vi "Dual Stream.vi"() -> ()   [LabVIEW 2016, in "Lab Streaming Layer.lvlib"]
uses:
  Lab Streaming Layer.lvlib
  Custom Controls/lsl_channel_format.ctl
panel:
  out "error out":errorcluster
  out "Array":dbl[][](array[numeric])
  out "Have Consumers":i32
  out "function return":i32
  in  "stop":bool
  out "source id":string
  out "nominal samplerate":dbl
  out "name":string
  out "channel bytes":i32
  out "channel count":i32
  out "xml":string
  out "version":i32
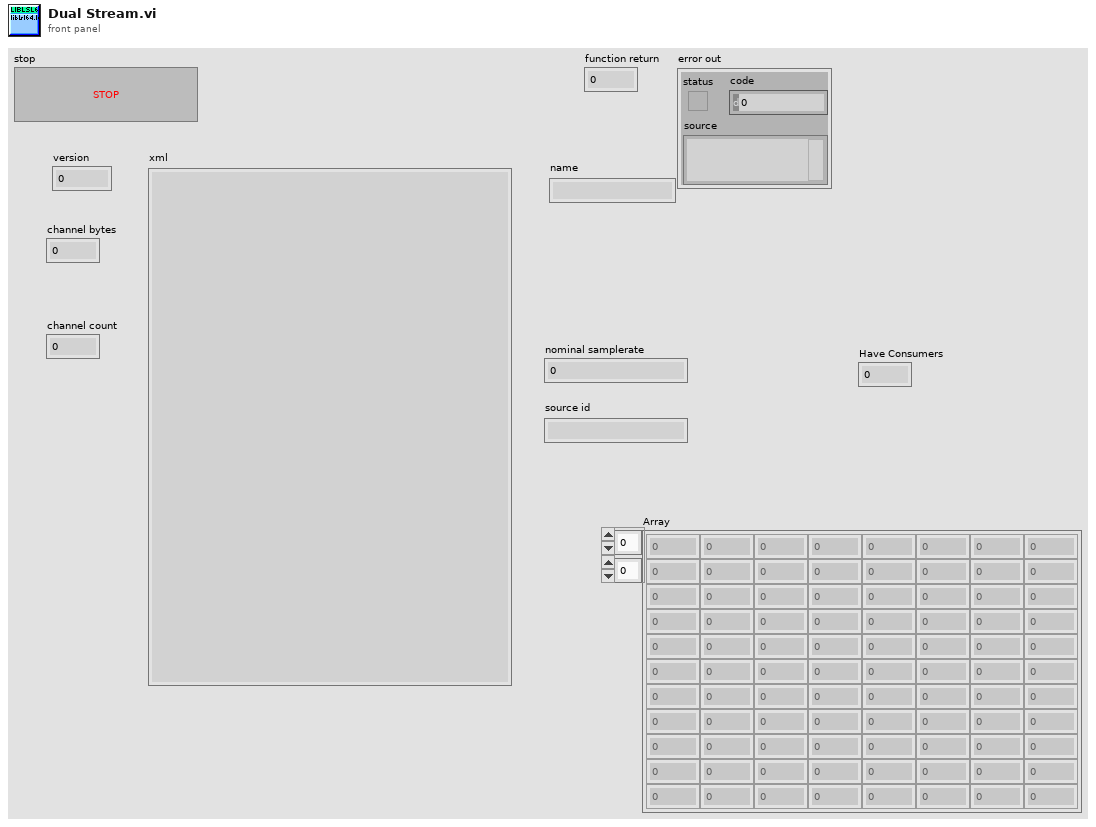
[diagram p1: front panel]
types:
  T1 = typedef "Lab Streaming Layer.lvlib/lsl_channel_format.ctl" = u32
  T2 = typedef "Lab Streaming Layer.lvlib/lsl_streaminfo.ctl" = u64
  T3 = typedef "Lab Streaming Layer.lvlib/lsl_outlet.ctl" = u64
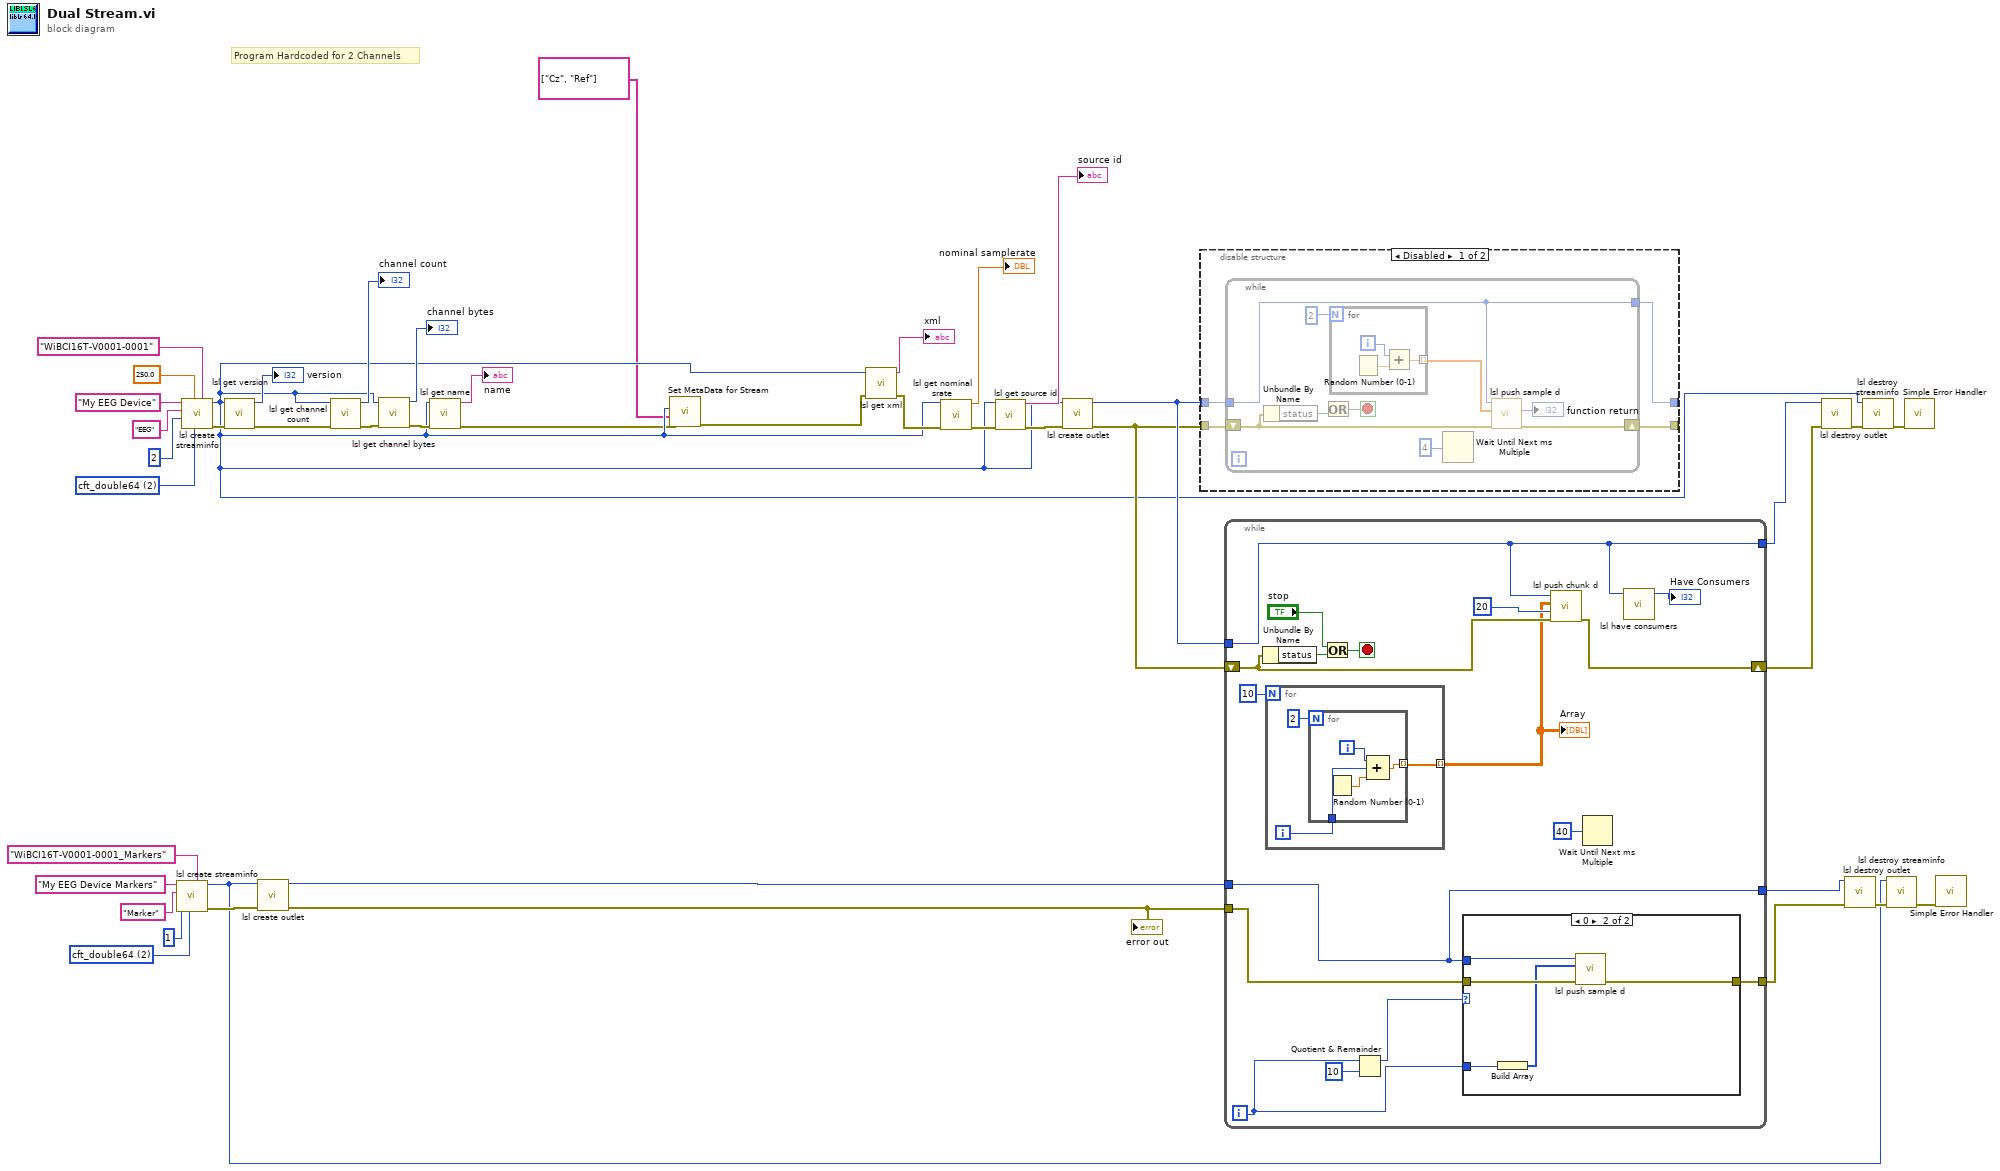
[diagram p0: block diagram]
diagram:
  w10 = T1 2 items=["cft_float32"=1, "cft_double64"=2, "cft_string"=3, "cft_int32"=4, "cft_int16"=5, "cft_int8"=6, "cft_int64"=7, "cft_undefined"=0] ("channel_format")
  w38 = T1 2 items=["cft_float32"=1, "cft_double64"=2, "cft_string"=3, "cft_int32"=4, "cft_int16"=5, "cft_int8"=6, "cft_int64"=7, "cft_undefined"=0] ("channel_format")
  # "Program Hardcoded for 2 Channels"
  n1 = call "lsl create streaminfo.vi"("source_id"="WiBCI16T-V0001-0001_Markers", "channel_format"=w10, "channel_count"=1, "type"="Marker", "name"="My EEG Device Markers") -> ("error out"=w9:errorcluster, "streaminfo"=w2:T2)  [unwired: 5 in]
  n2 = call "lsl create streaminfo.vi"("source_id"="WiBCI16T-V0001-0001", "channel_format"=w38, "samplingrate"=250.0, "channel_count"=2, "type"="EEG", "name"="My EEG Device") -> ("error out"=w37:errorcluster, "streaminfo"=w17:T2)  [unwired: 4 in]
  n3 = call "lsl get version.vi"("error in"=w37, "streaminfo"=w17) -> ("error out"=w20:errorcluster, "version"=→"version":i32)  [unwired: 8 in]
  n4 = call "lsl create outlet.vi"("error in (no error)"=w9, "streaminfo"=w2) -> ("error out"=w7:errorcluster, "outlet"=w8:T3)  [unwired: 8 in]
  "error out" <- w7
  n5 = call "lsl get channel count.vi"("error in (no error)"=w20, "streaminfo"=w17) -> ("error out"=w34:errorcluster, "channel count"=→"channel count":i32)  [unwired: 8 in]
  n6 = call "lsl get channel bytes.vi"("error in (no error)"=w34, "streaminfo"=w17) -> ("error out"=w32:errorcluster, "channel bytes"=→"channel bytes":i32)  [unwired: 8 in]
  n7 = call "lsl get name.vi"("error in (no error)"=w32, "streaminfo"=w17) -> ("error out"=w15:errorcluster, "name"=→"name":string)  [unwired: 8 in]
  n8 = call "Set MetaData for Stream.vi"("error in"=w15, "Ch Names"=string[] ["Cz", "Ref"], "streaminfo"=w17) -> ("error out"=w14:errorcluster)  [unwired: 8 in]
  n9 = call "lsl get xml.vi"("error in (no error)"=w14, "streaminfo"=w17) -> ("error out"=w18:errorcluster, "xml"=→"xml":string)  [unwired: 8 in]
  n10 = call "lsl get nominal srate.vi"("error in (no error)"=w18, "streaminfo"=w17) -> ("error out"=w29:errorcluster, "nominal samplerate"=→"nominal samplerate":dbl)  [unwired: 8 in]
  n11 = call "lsl get source id.vi"("error in (no error)"=w29, "streaminfo"=w17) -> ("error out"=w27:errorcluster, "source id"=→"source id":string)  [unwired: 8 in]
  n12 = call "lsl create outlet.vi"("error in (no error)"=w27, "streaminfo"=w17) -> ("error out"=w23:errorcluster, "outlet"=w24:T3)  [unwired: 8 in]
  n13 = disable-structure shown="Disabled" {
    disable-tunnel: w24 -> [w47 _]
    disable-tunnel: w23 -> [w46 _]
    disable-tunnel: [w45 _] -> _
    disable-tunnel: [w44 _] -> _
    frame Disabled {
      n14 = while {
        tunnel: w47 -> [w48]
        shift-right: [w52] -> w44
        shift-left: w46 -> [w53]
        tunnel: [w48] -> w45
        stop <- w54 stop-if-true
        n15 = Unbundle By Name(w53) -> ("status"=w55:bool)
        n16 = Or(y=w55) -> (x .or. y?=w54:bool)  [unwired: 1 in]
        n17 = for {
          N: 2 -> [_]
          tunnel: [w58] -> w51 mode=indexing
          i -> [w57]
          n18 = Random Number (0-1)() -> (number: 0 to 1=w59:dbl)
          n19 = Add(x=w57, y=w59) -> (x+y=w58:dbl)
        }
        n20 = Wait Until Next ms Multiple(millisecond multiple=u32 4) -> ()  [unwired: 1 out]
        n21 = call "lsl push sample d.vi"("error in (no error)"=w53, "data"=w51, "outlet"=w48) -> ("error out"=w52:errorcluster, "function return"=→"function return":i32)  [unwired: 7 in]
      }
    }
    frame Enabled {
    }
  }
  n22 = while {
    tunnel: w24 -> [w67]
    shift-right: [w72] -> w21
    shift-left: w23 -> [w73]
    tunnel: [w67] -> w22
    tunnel: w8 -> [w61]
    tunnel: w7 -> [w63]
    tunnel: [w61] -> w5
    tunnel: [w60] -> w4
    i -> [w62]
    stop <- w75 stop-if-true
    n23 = Unbundle By Name(w73) -> ("status"=w76:bool)
    n24 = for {
      N: 10 -> [_]
      tunnel: [w84] -> w68 mode=indexing
      i -> [w83]
      n25 = for {
        N: 2 -> [_]
        tunnel: [w89] -> w84 mode=indexing
        tunnel: w83 -> [w87]
        i -> [w88]
        n26 = Random Number (0-1)() -> (number: 0 to 1=w86:dbl)
        n27 = Compound Arithmetic op=ADD(w88, w87, w86) -> (w89:dbl)
      }
    }
    "Array" <- w68
    n28 = Or(x="stop", y=w76) -> (x .or. y?=w75:bool)
    n29 = Quotient & Remainder(x=w62, y=10) -> (x-y*floor(x/y)=w64:i32)  [unwired: 1 out]
    n30 = case shown="0" w64 {
      tunnel: w63 -> [w77 w81]
      tunnel: w61 -> [_ w82]
      tunnel: w62 -> [_ w80]
      tunnel: [w77 w78] -> w60
      frame 1, Default {
      }
      frame 0 {
        n31 = Build Array(w80) -> (w79:i32[])
        n32 = call "lsl push sample d.vi"("error in (no error)"=w81, "data"=w79, "outlet"=w82) -> ("error out"=w78:errorcluster)  [unwired: 7 in, 1 out]
      }
    }
    n33 = call "lsl push chunk d.vi"("error in (no error)"=w73, "data_elements"=i64 20, "data"=w68, "outlet"=w67) -> ("error out"=w72:errorcluster)  [unwired: 6 in, 1 out]
    n34 = Wait Until Next ms Multiple(millisecond multiple=u32 40) -> ()  [unwired: 1 out]
    n35 = call "lsl have consumers.vi"("outlet"=w67) -> ("Have Consumers"=→"Have Consumers":i32)  [unwired: 9 in, 1 out]
  }
  n36 = call "lsl destroy outlet.vi"("error in (no error)"=w21, "outlet"=w22) -> ("error out"=w25:errorcluster)  [unwired: 9 in]
  n37 = call "lsl destroy outlet.vi"("error in (no error)"=w4, "outlet"=w5) -> ("error out"=w6:errorcluster)  [unwired: 9 in]
  n38 = call "lsl destroy streaminfo.vi"("error in (no error)"=w25, "streaminfo"=w17) -> ("error out"=w26:errorcluster)  [unwired: 9 in]
  n39 = call "lsl destroy streaminfo.vi"("error in (no error)"=w6, "streaminfo"=w2) -> ("error out"=w3:errorcluster)  [unwired: 9 in]
  n40 = call <vilib>:"Simple Error Handler.vi"("error in (no error)"=w26) -> ()  [unwired: 4 in, 5 out]
  n41 = call <vilib>:"Simple Error Handler.vi"("error in (no error)"=w3) -> ()  [unwired: 4 in, 5 out]
